vi "Runtime Test.vi"() -> ()   [LabVIEW 2013, in "J1939 tests.lvlib"]
uses:
  J1939 tests.lvlib
  <vilib>/NI/Tag Bus/dictionary/full data dictionary.ctl
  module/execution/J1939 runtime.lvclass
  <vilib>/NI/Tag Bus Module Framework/channel/data tables.ctl
  <vilib>/NI/Tag Bus/dictionary table pair.ctl
  <vilib>/NI/Tag Bus/dictionary/data dictionary.lvclass
  <vilib>/NI/Tag Bus/table/data table.ctl
  module/configuration/J1939 configuration.lvclass/J1939 configuration.ctl
  <vilib>/NI/Tag Bus/table/data polymorphs/write many/write Singles.vi
  <vilib>/NI/Tag Bus/table/data polymorphs/read many/read Singles.vi
  module/configuration/Read XNET Settings.vi
  module/configuration/Read Lines.vi
  <vilib>/xnet/xnet.llb/XNET Create Session (Signal Output Single-point).vi
  module/execution/J1939 Claim With Address.vi
  <vilib>/xnet/xnet.llb/XNET Create Session (Signal Input Single-point).vi
  <vilib>/xnet/xnet.llb/XNET Write (Signal Single-point).vi
  <vilib>/xnet/xnet.llb/XNET Read (Signal Single-point).vi
  <vilib>/NI/Tag Bus Module Framework/channel/TBM channel.lvclass
  module/configuration/J1939 configuration.lvclass
  <vilib>/NI/Tag Bus/table/data table.lvlib
  <vilib>/NI/Tag Bus/tag bus.lvlib
panel:
  in  "Tag Bus Output":dbl[](array[knob])=[0.0, 0.0] caption="data" scale=0.0..50.0
  out "Tag Bus Input":dbl[](array[knob]) caption="data" scale=0.0..50.0
  out "dictionary":T1
  in  "stop":bool
  out "Signal Single Point Data":dbl[](array[knob]) caption="data" scale=0.0..50.0
  in  "Wirte Direct Can":dbl[](array[knob])=[0.0, 0.0] caption="data" scale=0.0..50.0
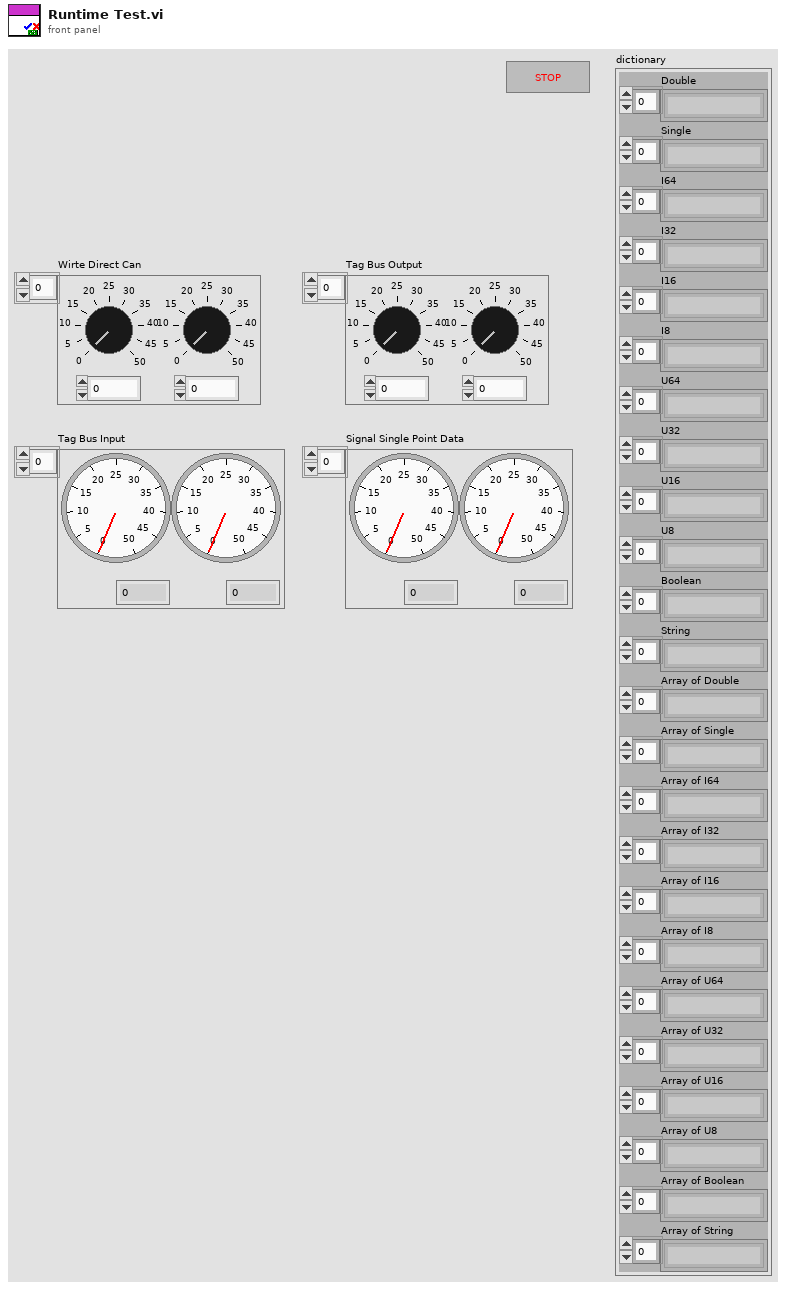
[diagram p1: front panel]
types:
  T1 = typedef "tag bus.lvlib/data dictionary.lvclass/full data dictionary.ctl" = cluster{"Double":string[], "Single":string[], "I64":string[], "I32":string[], "I16":string[], "I8":string[], "U64":string[], "U32":string[], "U16":string[], "U8":string[], "Boolean":string[], "String":string[], "Array of Double":string[], "Array of Single":string[], "Array of I64":string[], "Array of I32":string[], "Array of I16":string[], "Array of I8":string[], "Array of U64":string[], "Array of U32":string[], "Array of U16":string[], "Array of U8":string[], "Array of Boolean":string[], "Array of String":string[]}
  T2 = typedef "TBM channel.lvclass/data tables.ctl" = cluster{"input data":T3, "processing parameter":T3, "processing result":T3, "output data":T3}
  T3 = typedef "tag bus.lvlib/dictionary table pair.ctl" = cluster{"data dictionary":refnum<class "data dictionary.lvclass">, "data table":T4}
  T4 = typedef "tag bus.lvlib/data table.lvlib/data table.ctl" = cluster{"Double":dbl[], "Single":sgl[], "I64":i64[], "I32":i32[], "I16":i16[], "I8":i8[], "U64":u64[], "U32":u32[], "U16":u16[], "U8":u8[], "Boolean":bool[], "String":string[], "Array of Double":cluster{"DBL Array":dbl[]}[], "Array of Single":cluster{"SGL Array":sgl[]}[], "Array of I64":cluster{"I64 Array":i64[]}[], "Array of I32":cluster{"I32 Array":i32[]}[], "Array of I16":cluster{"I16 Array":i16[]}[], "Array of I8":cluster{"I8 Array":i8[]}[], "Array of U64":cluster{"U64 Array":u64[]}[], "Array of U32":cluster{"U32 Array":u32[]}[], "Array of U16":cluster{"U16 Array":u16[]}[], "Array of U8":cluster{"U8 Array":u8[]}[], "Array of Boolean":cluster{"Boolean Array":bool[]}[], "Array of String":cluster{"String Array":string[]}[]}
  T5 = typedef "J1939 configuration.lvclass/XNET Settings.ctl" = cluster{"Select Interface":refnum<k21>, "Node Address":u8, "Node Name":u64}
  T6 = typedef "J1939 configuration.lvclass/Line.ctl" = cluster{"channel":refnum<class "TBM channel.lvclass">, "XNET Signal":refnum<k21>}
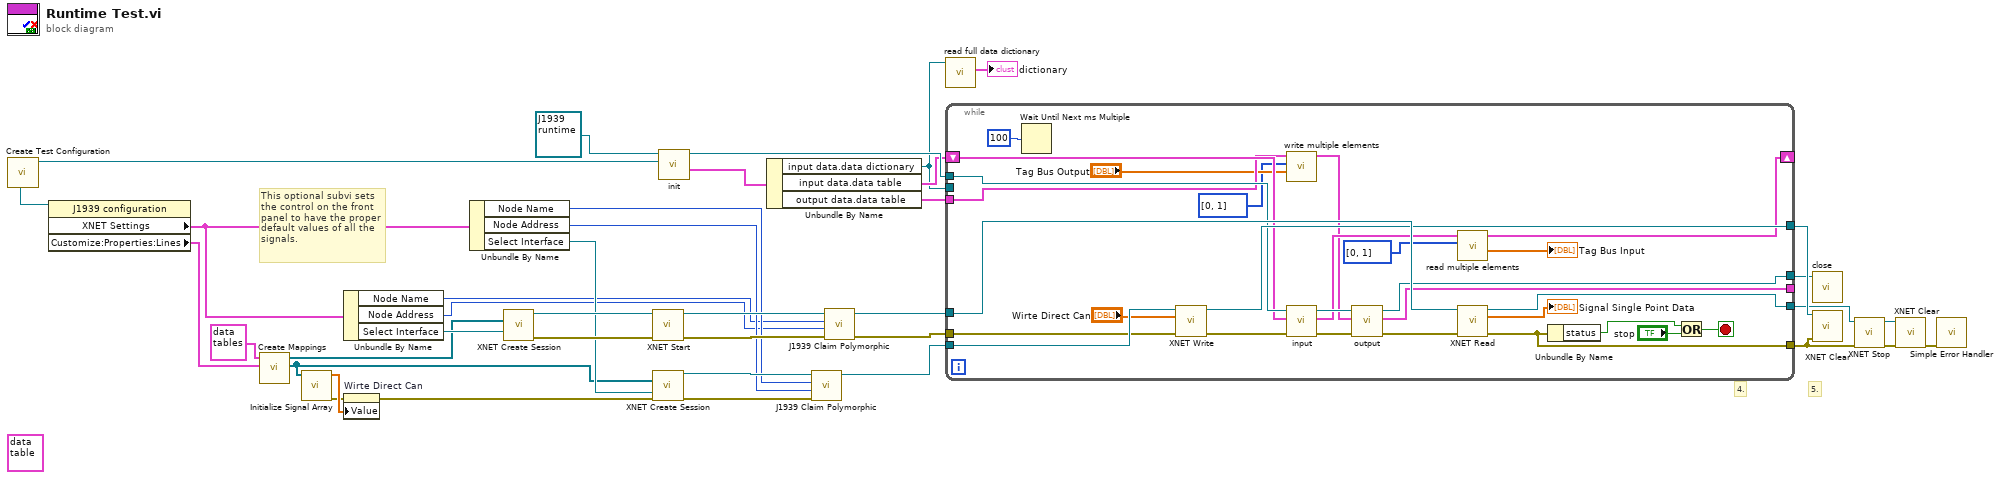
[diagram p0: block diagram]
diagram:
  (unwired) T4 {"Double"=[], "Single"=[], "I64"=[], "I32"=[], "I16"=[], "I8"=[], "U64"=[], "U32"=[], "U16"=[], "U8"=[], "Boolean"=[], "String"=[], "Array of Double"=[], "Array of Single"=[], "Array of I64"=[], "Array of I32"=[], "Array of I16"=[], "Array of I8"=[], "Array of U64"=[], "Array of U32"=[], "Array of U16"=[], "Array of U8"=[], "Array of Boolean"=[], "Array of String"=[]} ("data table")
  # "This optional subvi sets the control on the front panel to have the proper default values of all the signals."
  # "5."
  # "4."
  n1 = call "Create Test Configuration.vi"() -> ("Module Configuration"=w18:refnum<class "J1939 configuration.lvclass">, "Inverted Module Config"=w9:refnum<class "J1939 configuration.lvclass">)  [unwired: 5 in, 5 out]
  n2 = property class="J1939 configuration"(reference=w9) -> ("XNET Settings"=w1:T5, "Customize:Properties:Lines"=w17:T6[])  [unwired: 1 in, 2 out]
  n3 = call "Create Mappings.vi"("Lines"=w17, "data allocations"=T2 {"input data"={"data dictionary"=refnum, "data table"={"Double"=[], "Single"=[], "I64"=[], "I32"=[], "I16"=[], "I8"=[], "U64"=[], "U32"=[], "U16"=[], "U8"=[], "Boolean"=[], "String"=[], "Array of Double"=[], "Array of Single"=[], "Array of I64"=[], "Array of I32"=[], "Array of I16"=[], "Array of I8"=[], "Array of U64"=[], "Array of U32"=[], "Array of U16"=[], "Array of U8"=[], "Array of Boolean"=[], "Array of String"=[]}}, "processing parameter"={"data dictionary"=refnum, "data table"={"Double"=[], "Single"=[], "I64"=[], "I32"=[], "I16"=[], "I8"=[], "U64"=[], "U32"=[], "U16"=[], "U8"=[], "Boolean"=[], "String"=[], "Array of Double"=[], "Array of Single"=[], "Array of I64"=[], "Array of I32"=[], "Array of I16"=[], "Array of I8"=[], "Array of U64"=[], "Array of U32"=[], "Array of U16"=[], "Array of U8"=[], "Array of Boolean"=[], "Array of String"=[]}}, "processing result"={"data dictionary"=refnum, "data table"={"Double"=[], "Single"=[], "I64"=[], "I32"=[], "I16"=[], "I8"=[], "U64"=[], "U32"=[], "U16"=[], "U8"=[], "Boolean"=[], "String"=[], "Array of Double"=[], "Array of Single"=[], "Array of I64"=[], "Array of I32"=[], "Array of I16"=[], "Array of I8"=[], "Array of U64"=[], "Array of U32"=[], "Array of U16"=[], "Array of U8"=[], "Array of Boolean"=[], "Array of String"=[]}}, "output data"={"data dictionary"=refnum, "data table"={"Double"=[], "Single"=[], "I64"=[], "I32"=[], "I16"=[], "I8"=[], "U64"=[], "U32"=[], "U16"=[], "U8"=[], "Boolean"=[], "String"=[], "Array of Double"=[], "Array of Single"=[], "Array of I64"=[], "Array of I32"=[], "Array of I16"=[], "Array of I8"=[], "Array of U64"=[], "Array of U32"=[], "Array of U16"=[], "Array of U8"=[], "Array of Boolean"=[], "Array of String"=[]}}}) -> ("Output Singals"=w16:refnum<k21>[], "Input Singals"=w15:refnum<k21>[])  [unwired: 6 in, 2 out]
  n4 = call "Initialize Signal Array.vi"("signal list"=w16) -> ("error out"=w31:errorcluster, "Array"=w32:dbl[])  [unwired: 1 in, 6 out]
  n5 = Unbundle By Name(w1) -> ("Node Name"=w23:u64, "Node Address"=w24:u8, "Select Interface"=w22:refnum<k21>)
  n6 = property on="Wirte Direct Can" class="Arr (strict)"(error in=w31, "Value"=w32) -> (error out=w30:errorcluster)  [unwired: 1 in, 1 out]
  n7 = Unbundle By Name(w1) -> ("Node Name"=w27:u64, "Node Address"=w26:u8, "Select Interface"=w25:refnum<k21>)
  n8 = call-poly <vilib>:"XNET Create Session.vi"("signal list"=w15, "interface"=w22) -> ("session out"=w39:refnum<k21>, "error out"=w38:errorcluster)  [unwired: 1 in, 11 out]
  n9 = call <vilib>:"XNET Start.vi"("session in"=w39, "error in (no error)"=w38) -> ("session out"=w36:refnum<k21>, "error out"=w35:errorcluster)  [unwired: 12 in]
  n10 = call-poly <vilib>:"XNET Create Session.vi"("signal list"=w16, "interface"=w25, "error in (no error)"=w30) -> ("session out"=w29:refnum<k21>, "error out"=w28:errorcluster)  [unwired: 11 out]
  n11 = call-dynamic "init.vi"("TBM module configuration in"=w18, "J1939 runtime in"=refnum<class "J1939 runtime.lvclass"> refnum ("J1939 runtime")) -> ("data allocations"=w12:T2, "J1939 runtime out"=w14:refnum<class "J1939 runtime.lvclass">)  [unwired: 6 in, 2 out]
  n12 = Unbundle By Name(w12) -> ("input data.data dictionary"=w7:refnum<class "data dictionary.lvclass">, "input data.data table"=w11:T4, "output data.data table"=w10:T4)
  n13 = call-poly "J1939 Claim Polymorphic.vi"("error in (no error)"=w28, "SAE J1939:Node Address"=w26, "SAE J1939:Node Name"=w27, "XNET Session"=w29) -> ("XNET Session Out"=w21:refnum<k21>)  [unwired: 5 in, 2 out]
  n14 = call-poly "J1939 Claim Polymorphic.vi"("error in (no error)"=w35, "SAE J1939:Node Address"=w24, "SAE J1939:Node Name"=w23, "XNET Session"=w36) -> ("error out"=w34:errorcluster, "XNET Session Out"=w33:refnum<k21>)  [unwired: 5 in, 1 out]
  n15 = call <vilib>:"read full data dictionary.vi"("data dictionary in"=w7) -> ("dictionary"=→"dictionary":T1)  [unwired: 8 in, 2 out]
  n16 = while {
    tunnel: [w47] -> w4
    tunnel: w33 -> [w64]
    tunnel: w34 -> [w60]
    tunnel: [w62] -> w5
    tunnel: w21 -> [w61]
    tunnel: [w59] -> w20
    tunnel: w14 -> [w58]
    shift-right: [w44] -> _
    shift-left: w11 -> [w57]
    tunnel: [w55] -> w13
    tunnel: [w54] -> _
    tunnel: w10 -> [w53]
    tunnel: w7 -> [_]
    stop <- w65 stop-if-true
    n17 = Wait Until Next ms Multiple(millisecond multiple=u32 100 ("milliseconds to wait")) -> ()  [unwired: 1 out]
    n18 = call-poly <vilib>:"XNET Write.vi"("session in"=w61, "data"="Wirte Direct Can", "error in (no error)"=w60) -> ("session out"=w59:refnum<k21>, "error out"=w50:errorcluster)  [unwired: 11 out]
    n19 = call-poly <vilib>:"write multiple elements.vi"("values"="Tag Bus Output", "indices"=i32[] [0, 1], "data table in"=w53) -> ("data table out"=w42:T4)  [unwired: 8 in]
    n20 = call-dynamic "input.vi"("error in"=w50, "data table in"=w57, "J1939 runtime in"=w58) -> ("error out"=w49:errorcluster, "data table out"=w45:T4, "J1939 runtime out"=w56:refnum<class "J1939 runtime.lvclass">)  [unwired: 6 in]
    n21 = call-dynamic "output.vi"("error in"=w49, "data table in"=w42, "J1939 runtime in"=w56) -> ("error out"=w48:errorcluster, "data table out"=w54:T4, "J1939 runtime out"=w55:refnum<class "J1939 runtime.lvclass">)  [unwired: 6 in]
    n22 = call-poly <vilib>:"read multiple elements.vi"("indices"=i32[] [0, 1], "data table in"=w45) -> ("values"=→"Tag Bus Input":sgl[], "data table out"=w44:T4)  [unwired: 8 in]
    n23 = call-poly <vilib>:"XNET Read.vi"("session in"=w64, "error in (no error)"=w48) -> ("session out"=w62:refnum<k21>, "data"=→"Signal Single Point Data":dbl[], "error out"=w47:errorcluster)  [unwired: 11 out]
    n24 = Unbundle By Name(w47) -> ("status"=w67:bool)
    n25 = Or(x=w67, y="stop") -> (x .or. y?=w65:bool)
  }
  n26 = call-dynamic "close.vi"("J1939 runtime in"=w13) -> ()  [unwired: 10 in, 1 out]
  n27 = call <vilib>:"XNET Clear.vi"("session in"=w20, "error in (no error)"=w4) -> ()  [unwired: 13 in, 1 out]
  n28 = call <vilib>:"XNET Stop.vi"("session in"=w5, "error in (no error)"=w4) -> ("session out"=w2:refnum<k21>, "error out"=w3:errorcluster)  [unwired: 12 in]
  n29 = call <vilib>:"XNET Clear.vi"("session in"=w2, "error in (no error)"=w3) -> ("error out"=w37:errorcluster)  [unwired: 13 in]
  n30 = call <vilib>:"Simple Error Handler.vi"("error in (no error)"=w37) -> ()  [unwired: 1 in, 8 out]
